vi "Measure Capacitance w RFSwitch.vi"(2 "VNAs Measurement Parameters":T1, 8 "error in (no error)":errorcluster, 9 "Measurement Id":string="CFree", 11 "Semiconductor Module Context":T2) -> (0 "error out":errorcluster, 1 "Multisite Cap Data":dbl[][](array[numeric]), 3 "Semiconductor Module Context Out":T2)   [LabVIEW 2013]
uses:
  <vilib>/NI_TestStand_SemiconductorModule/NI_TestStand_Semiconductor_Module.lvlibp/PinMap/General/SemiconductorModuleContext.ctl
  VNA/VNAs Measurement Parameters.ctl
  <vilib>/NI_TestStand_SemiconductorModule/NI_TestStand_Semiconductor_Module.lvlibp
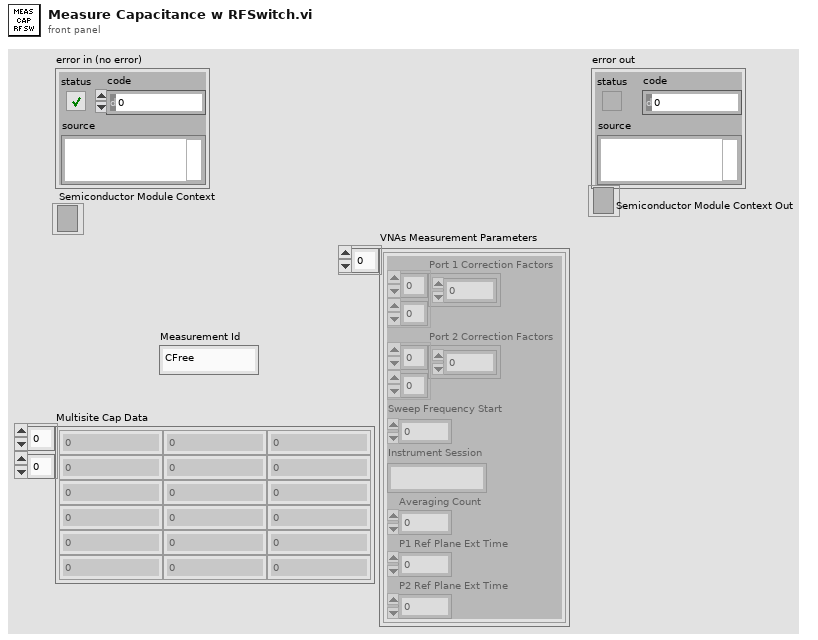
[diagram p1: front panel]
types:
  T1 = typedef "VNAs Measurement Parameters.ctl" = cluster{"Port 1 Correction Factors":cdb[][], "Port 2 Correction Factors":cdb[][], "Sweep Frequency Start":dbl, "Instrument Session":string, "Averaging Count":i32, "P1 Ref Plane Ext Time":dbl, "P2 Ref Plane Ext Time":dbl}[]
  T2 = typedef "NI_TestStand_Semiconductor_Module.lvlibp/SemiconductorModuleContext.ctl" = refnum<k7>
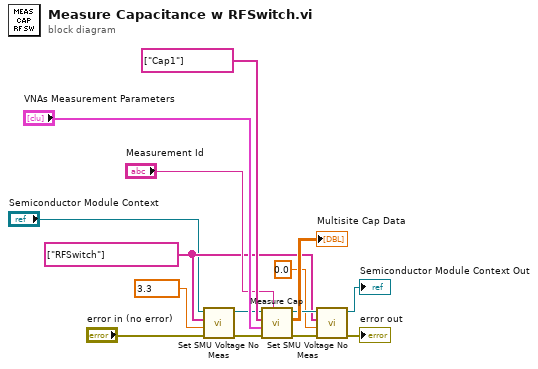
[diagram p0: block diagram]
diagram:
  w7 = string[] ["RFSwitch"] ("RFSwitch Pin")
  n1 = call "Set SMU Voltage No Meas.vi"("error in (no error)"="error in (no error)", "VDD voltage level"=3.3 ("RFSwitch_V1_level"), "Pins"=w7, "Semiconductor Module Context"="Semiconductor Module Context") -> ("error out"=w11:errorcluster, "Semiconductor Module Context Out"=w8:T2)  [unwired: 5 in, 1 out]
  n2 = call "Measure Cap.vi"("Measurement Id"="Measurement Id", "error in (no error)"=w11, "VNAs Measurement Parameters"="VNAs Measurement Parameters", "Pins"=string[] ["Cap1"] ("Capacitance Pins"), "Semiconductor Module Context"=w8) -> ("error out"=w10:errorcluster, "Multisite Cap Data"=→"Multisite Cap Data":dbl[][], "Semiconductor Module Context Out"=w9:T2)  [unwired: 4 in]
  n3 = call "Set SMU Voltage No Meas.vi"("error in (no error)"=w10, "VDD voltage level"=0.0, "Pins"=w7, "Semiconductor Module Context"=w9) -> ("error out"=→"error out":errorcluster, "Semiconductor Module Context Out"=→"Semiconductor Module Context Out":T2)  [unwired: 5 in, 1 out]
